vi "Pre Launch Init.vi"(11 "Mag Lab Root in":refnum<class "Mag Lab Root.lvclass">) -> (0 "error out":errorcluster, 3 "Mag Lab Root out":refnum<class "Mag Lab Root.lvclass">)   [LabVIEW 2015, in "Mag Lab Root.lvclass"]
doc: "(<B>Filename</B>: Actor Framework.lvlib:Actor.lvclass:Pre Launch Init.vi)\n\nDefines behavior that occurs after the Launch Nested Actor method is invoked but before the actor's Actor Core method begins running.\n\nBy default, this method does nothing. A descendant class may override it to define behavior."
uses:
  Mag Lab Root.lvclass
  Mag Lab Root.lvclass/Mag Lab Root.ctl
  <vilib>/ActorFramework/Actor/Actor.lvclass
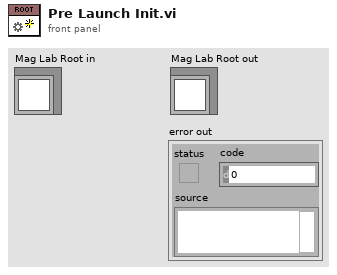
[diagram p1: front panel]
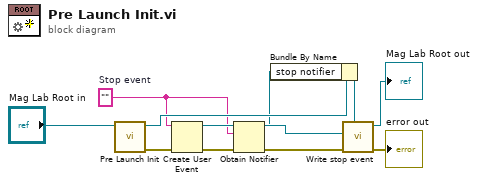
[diagram p0: block diagram]
diagram:
  w3 = ""  # Stop event
  n1 = call-parent "Pre Launch Init.vi"("Actor in"="Mag Lab Root in") -> ("error out"=w10:errorcluster, "Actor out"=w6:refnum<class "Mag Lab Root.lvclass">)  [unwired: 9 in]
  n2 = Create User Event(user event datatype=w3, error in=w10) -> (user event=w7:refnum<user-event>, error out=w9:errorcluster)
  n3 = Obtain Notifier(notification data type=w3, error in (no error)=w9) -> (notifier out=w1:refnum<notifier>, error out=w4:errorcluster)  [unwired: 2 in, 1 out]
  n4 = Bundle By Name(cluster=w6, "stop notifier"=w1) -> (w2:refnum<class "Mag Lab Root.lvclass">)
  n5 = call "Write stop event.vi"("error in (no error)"=w4, "stop event"=w7, "Mag Lab Root in"=w2) -> ("error out"=→"error out":errorcluster, "Mag Lab Root out"=→"Mag Lab Root out":refnum<class "Mag Lab Root.lvclass">)  [unwired: 7 in]
